vi "Test Rotation Shift.vi"() -> ()   [LabVIEW 2020]
uses:
  Labview Library/Libraries/Basic Experiment/AutoTrace Element Result.ctl
  Labview Library/Libraries/Shift_Correction/Libraries/Shift_Correction/Marker Trace Mode.ctl
  <vilib>/Analysis/coordinate.llb/3D Coordinate Conversion (Scalar).vi
  <vilib>/Utility/file.llb/Read Delimited Spreadsheet (string).vi
  Labview Library/Libraries/Read TDMS Data/Library/Read TDMS Data.lvlib
  Labview Library/Libraries/Basic Experiment/Basic Experiment.lvlib
  Labview Library/Libraries/Shift_Correction/Libraries/Shift_Correction/Shift_Correction.lvlib
  <vilib>/Analysis/NI_AALPro.lvlib
panel:
  out "Amp Diff Array":dbl[](array[numeric])
  out "Angle Diff Array":dbl[](array[numeric]) format="%#.3g"
  out "Amp Difference":dbl
  out "Angle Difference (deg)":dbl
  out "AutoTrace Result":T1={"Pure Count"=18402.069978803433, "BackGround"=0.0, "AutoTrace File Path"=path "G:/Raw Data/AutoFocus/Z TDMS/2024-03/AF Z 2024-03-07_233436.png", "Light Spot Pos"=[76.30805206, 189.9241638, 65.24230408]}
  in  "ColorCenter List Path":path=path "G:/Exp_Log/2024_02_12_ChargeDetection2/Accurate_LightSpot.csv"
  out "Table":string[][](array[string])
  in  "Index":u32[](array[numeric])
  # "The shapes of some lightspot are bad. for now we can just watch the Confocal UI to check this. In the future we all save the picture of Trace to Specific Location to let you check."
  # "You should further substract this difference in \nyour Map Angle Correction Setting."
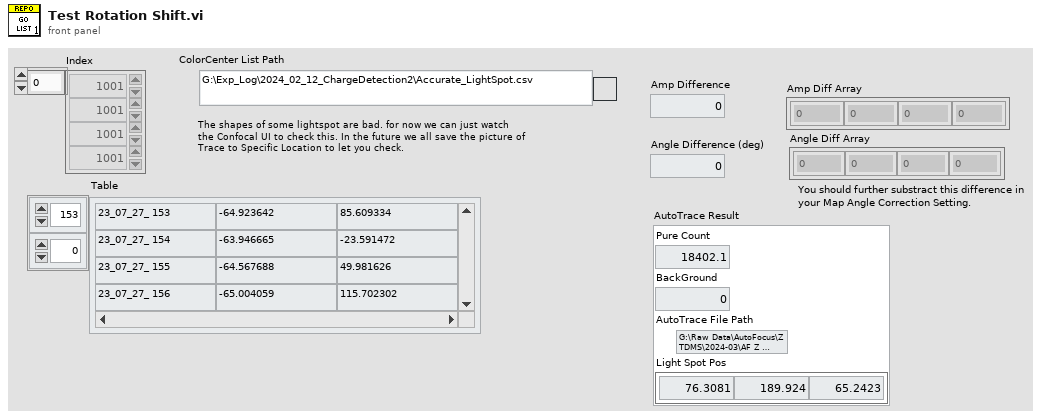
[diagram p1: front panel]
types:
  T1 = typedef "Basic Experiment.lvlib/AutoTrace Element Result.ctl" = cluster{"Pure Count":dbl, "BackGround":dbl, "AutoTrace File Path":path, "Light Spot Pos":dbl[]}
  T2 = typedef "Shift_Correction.lvlib/Marker Trace Mode.ctl" = enum16{"Trace Now", "Do Not Trace", "Auto"}
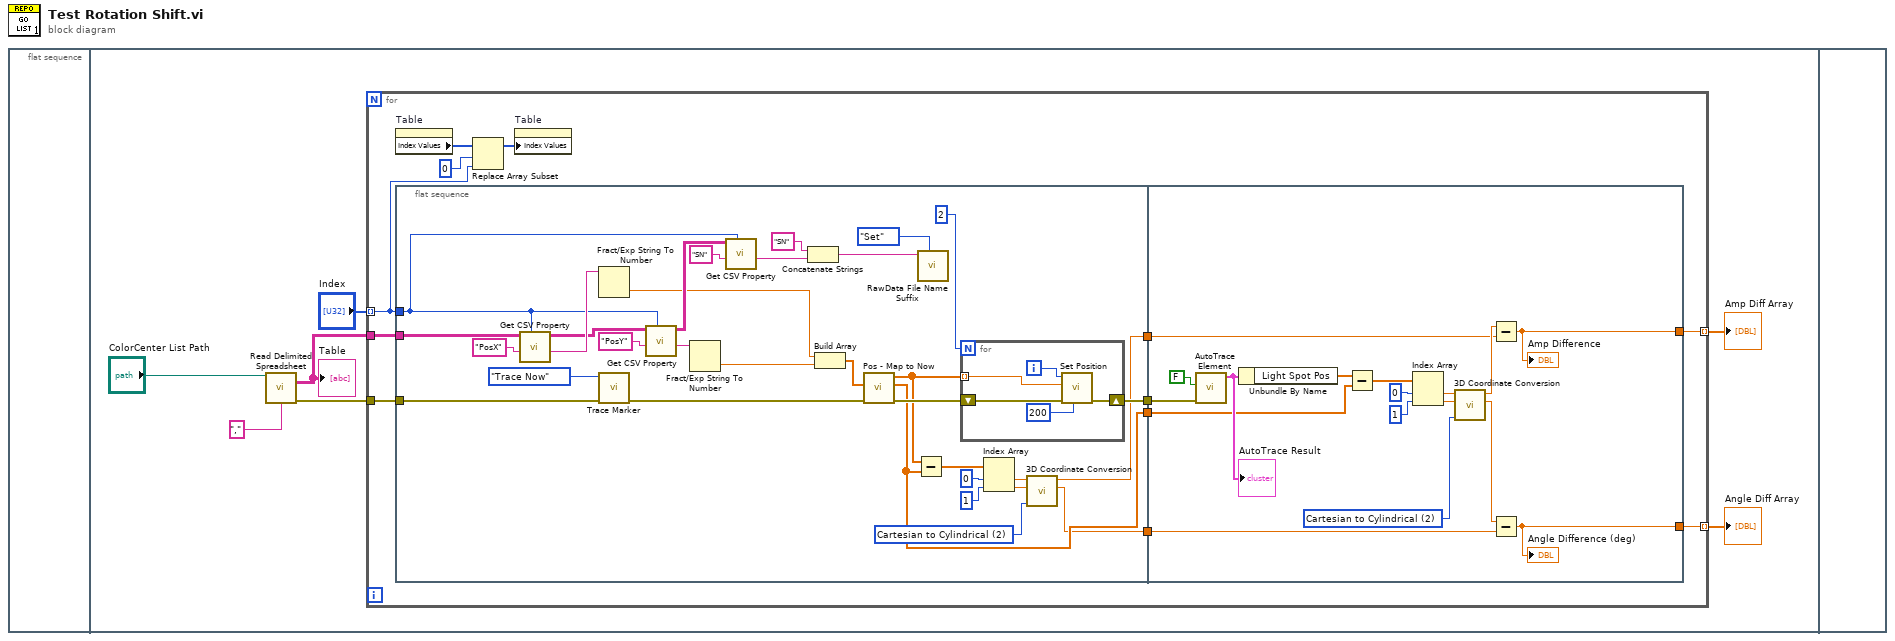
[diagram p0: block diagram]
diagram:
  n1 = flat-sequence {
    frame #0 {
    }
    frame #1 {
      n2 = call-poly <vilib>:"Read Delimited Spreadsheet.vi"("file path (dialog if empty)"="ColorCenter List Path", "delimiter (\\t)"="," ("delimiter (\\t)")) -> ("all rows"=w4:string[][], "error out"=w6:errorcluster)  [unwired: 8 in, 4 out]
      "Table" <- w4
      n3 = for {
        tunnel: w6 -> [w15]
        tunnel: w4 -> [w14]
        tunnel: "Index" -> [w10] mode=indexing
        tunnel: [w9] -> w1 mode=indexing
        tunnel: [w8] -> w2 mode=indexing
        n4 = property on="Table" class="Arr (strict)"() -> ("Index Values"=w13:u32[])  [unwired: 2 in, 2 out]
        n5 = flat-sequence {
          tunnel: [w33] -> w19
          tunnel: w15 -> [w21]
          tunnel: w10 -> [w43]
          tunnel: w14 -> [w50]
          tunnel: [w25] -> w18
          tunnel: [w24] -> w17
          tunnel: [w23] -> w16
          tunnel: w19 -> [w73]
          tunnel: w18 -> [w69]
          tunnel: w17 -> [w61]
          tunnel: w16 -> [w59]
          tunnel: [w58] -> w9
          tunnel: [w57] -> w8
          frame #0 {
            w26 = u16 2 items=["Cartesian to Spherical", "Spherical to Cartesian", "Cartesian to Cylindrical", "Cylindrical to Cartesian", "Spherical to Cylindrical", "Cylindrical to Spherical"] ("conversion type")
            n6 = call "Get CSV Property.vi"("Index"=w43, "Property Name"="PosX", "csv"=w50) -> ("Property value"=w49:string, "csv output"=w48:string[][])  [unwired: 7 in]
            n7 = Fract/Exp String To Number(string=w49) -> (number=w38:dbl)  [unwired: 3 in, 1 out]
            n8 = call "Trace Marker.vi"("error in"=w21, "Marker Trace Mode"=Marker_Trace_Mode."Trace Now") -> ("error out"=w20:errorcluster)  [unwired: 8 in, 1 out]
            n9 = call "Get CSV Property.vi"("Index"=w43, "Property Name"="PosY", "csv"=w48) -> ("Property value"=w47:string, "csv output"=w45:string[][])  [unwired: 7 in]
            n10 = Fract/Exp String To Number(string=w47) -> (number=w37:dbl)  [unwired: 3 in, 1 out]
            n11 = call "Get CSV Property.vi"("Index"=w43, "Property Name"="SN", "csv"=w45) -> ("Property value"=w40:string)  [unwired: 7 in, 1 out]
            n12 = Concatenate Strings("SN" ("string"), w40) -> (w39:string)
            n13 = Build Array(w38, w37) -> (w35:dbl[])
            n14 = call "Pos - Map to Now.vi"("error in"=w20, "Goal Map Position"=w35) -> ("error out"=w34:errorcluster, "Marker Position Now"=w25:dbl[], "Goal Now Position"=w30:dbl[])  [unwired: 6 in, 1 out]
            n15 = Subtract(x=w30, y=w25) -> (x-y=w29:dbl[])
            n16 = call "RawData File Name Suffix.vi"("Mode"=enum16{"Set", "Get"}."Set", "Suffix"=w39) -> ()  [unwired: 9 in, 1 out]
            n17 = for {
              N: 2 -> [_]
              tunnel: w30 -> [w56] mode=indexing
              shift-right: [w54] -> w33
              shift-left: w34 -> [w53]
              i -> [w55]
              n18 = call "Set Position.vi"("Idle After Moving (ms)"=200, "error in"=w53, "Position"=w56, "Axis"=w55) -> ("error out"=w54:errorcluster)  [unwired: 7 in]
            }
            n19 = Index Array(array=w29, index #1=0 ("index"), index #2=1 ("index")) -> (element #1=w28:dbl, element #2=w27:dbl)
            n20 = call-poly <vilib>:"3D Coordinate Conversion.vi"("conversion type"=w26, "axis 2"=w27, "axis 1"=w28) -> ("axis 2 out"=w23:dbl, "axis 1 out"=w24:dbl)  [unwired: 5 in, 2 out]
          }
          frame #1 {
            w68 = u16 2 items=["Cartesian to Spherical", "Spherical to Cartesian", "Cartesian to Cylindrical", "Cylindrical to Cartesian", "Spherical to Cylindrical", "Cylindrical to Spherical"] ("conversion type")
            n21 = call "AutoTrace Element.vi"("error in (no error)"=w73, "Need Correct Count?(T)"=FALSE) -> ("AutoTrace Result"=w71:T1)  [unwired: 8 in, 1 out]
            "AutoTrace Result" <- w71
            n22 = Unbundle By Name(w71) -> ("Light Spot Pos"=w70:dbl[])
            n23 = Subtract(x=w70, y=w69) -> (x-y=w63:dbl[])
            n24 = Index Array(array=w63, index #1=0 ("index"), index #2=1 ("index")) -> (element #1=w66:dbl, element #2=w67:dbl)
            n25 = call-poly <vilib>:"3D Coordinate Conversion.vi"("conversion type"=w68, "axis 2"=w67, "axis 1"=w66) -> ("axis 2 out"=w60:dbl, "axis 1 out"=w62:dbl)  [unwired: 5 in, 2 out]
            n26 = Subtract(x=w62, y=w61) -> (x-y=w58:dbl)
            "Amp Difference" <- w58
            n27 = Subtract(x=w60, y=w59) -> (x-y=w57:dbl)
            "Angle Difference (deg)" <- w57
          }
        }
        n28 = Replace Array Subset(array=w13, new element=w10, index=0) -> (w11:u32[])
        n29 = property on="Table" class="Arr (strict)"("Index Values"=w11) -> ()  [unwired: 2 in, 2 out]
      }
      "Angle Diff Array" <- w2
      "Amp Diff Array" <- w1
    }
    frame #2 {
    }
  }
